vi "XNET.Create.Signal.vi"(8 "error in":errorcluster, 10 "Signal":T1 {"Byte Order" items=["Little Endian", "Big Endian"]; "Data Type" items=["Signed", "Unsigned", "IEEE Float"]}, 11 "frame in":refnum<k21>) -> (0 "error out":errorcluster, 2 "signal out":refnum<k21>, 3 "frame out":refnum<k21>)   [LabVIEW 2024, in "Diagnostics Addon Shared.lvlib"]
uses:
  Diagnostics Addon Shared.lvlib
  Types/Signal.ctl
  <vilib>/xnet/xnet.llb/XNET Database Create (Signal).vi
  <resource>/objmgr/xnet.rc
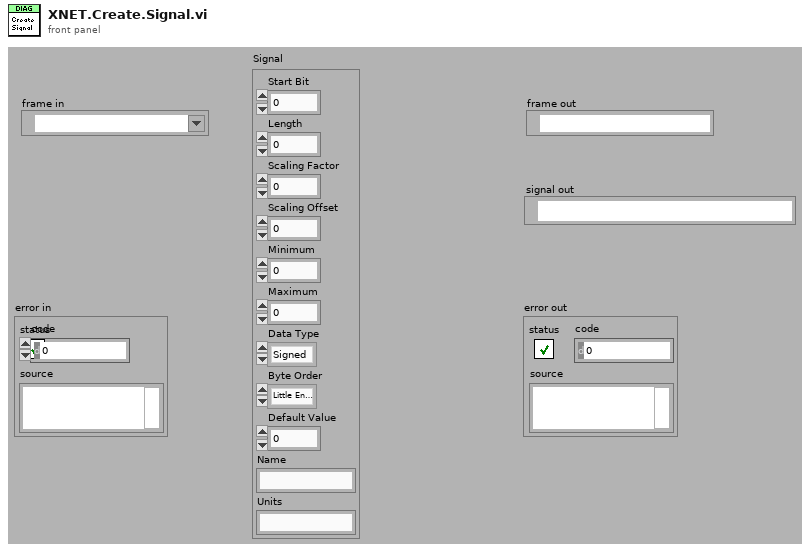
[diagram p1: front panel]
types:
  T1 = typedef "Diagnostics Addon Shared.lvlib/Signal.ctl" = cluster{"Start Bit":u32, "Length":u32, "Scaling Factor":dbl, "Scaling Offset":dbl, "Minimum":dbl, "Maximum":dbl, "Data Type":u32, "Byte Order":u32, "Default Value":dbl, "Name":string, "Units":string}
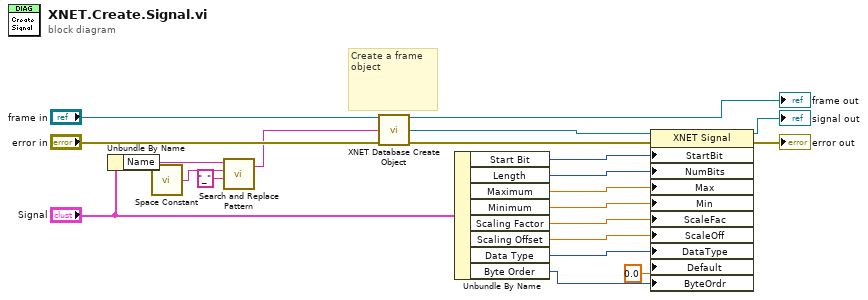
[diagram p0: block diagram]
diagram:
  # "Create a frame object"
  n1 = Unbundle By Name("Signal") -> ("Name"=w14:string)
  n2 = call <vilib>:"Space Constant.vi"() -> ("String"=w13:string)
  n3 = call <vilib>:"Search and Replace Pattern.vi"("string"=w14, "regular expression (\"\")"=w13, "replace string (\"\")"="_" ("replace string (\"\")")) -> ("result string"=w10:string)  [unwired: 2 in, 1 out]
  n4 = call-poly <vilib>:"XNET Database Create Object.vi"("frame in"="frame in", "signal name"=w10, "error in (no error)"="error in") -> ("frame out"=→"frame out":refnum<k21>, "signal out"=w18:refnum<k21>, "error out"=w20:errorcluster)  [unwired: 10 in]
  n5 = Unbundle By Name("Signal") -> ("Start Bit"=w9:u32, "Length"=w8:u32, "Maximum"=w7:dbl, "Minimum"=w6:dbl, "Scaling Factor"=w5:dbl, "Scaling Offset"=w4:dbl, "Data Type"=w3:u32, "Byte Order"=w2:u32)
  n6 = property class="XNET Signal"(reference=w18, error in=w20, "StartBit"=w9, "NumBits"=w8, "Max"=w7, "Min"=w6, "ScaleFac"=w5, "ScaleOff"=w4, "DataType"=w3, "Default"=0.0 ("Default Value"), "ByteOrdr"=w2) -> (reference out=→"signal out":refnum<k21>, error out=→"error out":errorcluster)
